vi "Host Example.vi"() -> ()   [LabVIEW 2015]
uses:
  Engine/Types/Buffered RT Instrument Command.ctl
  Shared/Types/Response Wait Type.ctl
  Engine/Types/Buffered RT Instrument Request.ctl
  Instrument CD Host API.lvlib
  Shared/Instrument Addon Shared.lvlib
  Engine/Instrument Addon Engine.lvlib
panel:
  out "Timed Out?":bool
  out "Response":T1
  in  "Command Parameters":T2
  out "error out":errorcluster
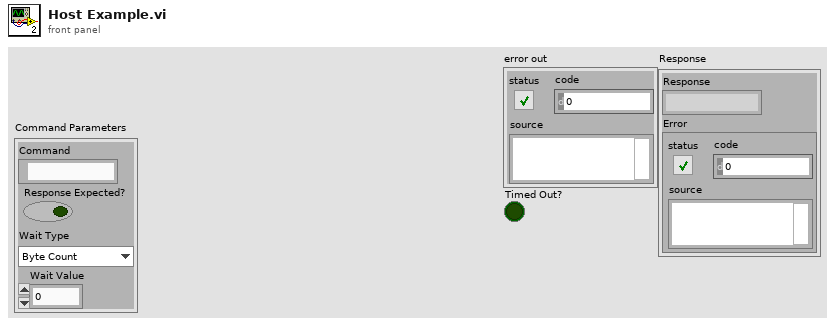
[diagram p1: front panel]
types:
  T1 = typedef "Instrument Addon Engine.lvlib/Buffered RT Instrument Request.ctl" = cluster{"Response":string, "Error":errorcluster}
  T2 = typedef "Instrument Addon Engine.lvlib/Buffered RT Instrument Command.ctl" = cluster{"Command":string, "Response Expected?":bool, "Wait Type":T3, "Wait Value":dbl}
  T3 = typedef "Instrument Addon Shared.lvlib/Response Wait Type.ctl" = enum16{"Byte Count", "Wait sec"}
  T4 = typedef "NI STM.lvlib/TCP Connection Info.ctl" = cluster{"connection ID":refnum<k5>, "meta data":T5[]}
  T5 = typedef "NI STM.lvlib/MetaDataElement.ctl" = string
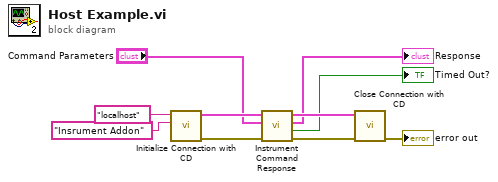
[diagram p0: block diagram]
diagram:
  n1 = call "Initialize Connection with CD.vi"("TCP Service"="Insrument Addon", "IP Address"="localhost") -> ("error out"=w9:errorcluster, "connection info out"=w10:T4)  [unwired: 8 in]
  n2 = call "Instrument Command Response.vi"("error in (no error)"=w9, "Command Parameters"="Command Parameters", "connection info"=w10) -> ("error out"=w8:errorcluster, "Timed Out?"=→"Timed Out?":bool, "Response"=→"Response":T1, "connection info"=w7:T4)  [unwired: 5 in]
  n3 = call "Close Connection with CD.vi"("error in"=w8, "connection info"=w7) -> ("error out"=→"error out":errorcluster)  [unwired: 9 in]
